vi "Requests.vi"(8 "error in (no error)":errorcluster, 9 "write enable":bool=TRUE, 11 "SMSD in":refnum<class "SMSD-DI.lvclass">) -> (0 "error out":errorcluster, 3 "SMSD out":refnum<class "SMSD-DI.lvclass">)   [LabVIEW 2019, in "SMSD-DI.lvclass"]
uses:
  SMSD-DI.lvclass
  D:/my_projects/projects/Algorithms/Labview/19/Modbus/MB_TCP2/MB_TCP.lvclass
  D:/my_projects/projects/Algorithms/Labview/19/Modbus/MB_TCP2/SMSD/SMSD.lvclass
  MB_TCP.lvclass/MB_TCP.ctl
  Ctl/ERROR_OR_COMMANT_Type.ctl
  SMSD.lvclass/SMSD.ctl
  NI_modbus_upd/TCP/TCP.lvclass/TCP.ctl
  SMSD_cmd_format.vi
  NI_modbus_upd/TCP/Protocol Read.vi
  NI_modbus_upd/TCP/Protocol Write.vi
  Data Access/Read TCP.vi
  SMSD_cmd_Data_format.vi
  SMSD_LAN_COMMAND.vi
  <vilib>/Utility/error.llb/Clear Errors.vi
  SMSD.lvclass
  NI_modbus_upd/TCP/TCP.lvclass
  ICPCON Registers/ICPCON Registers.lvlib
  MB_TCP.lvclass
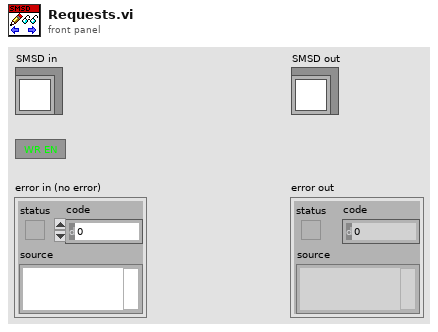
[diagram p1: front panel]
types:
  T1 = enum8{"CMD_PowerSTEP01_END", "CMD_PowerSTEP01_GET_SPEED", "CMD_PowerSTEP01_STATUS_IN_EVENT", "CMD_PowerSTEP01_SET_MODE", "CMD_PowerSTEP01_GET_MODE", "CMD_PowerSTEP01_SET_MIN_SPEED", "CMD_PowerSTEP01_SET_MAX_SPEED", "CMD_PowerSTEP01_SET_ACC", "CMD_PowerSTEP01_SET_DEC", "CMD_PowerSTEP01_SET_FS_SPEED", "CMD_PowerSTEP01_SET_MASK_EVENT", "CMD_PowerSTEP01_GET_ABS_POS", "CMD_PowerSTEP01_GET_EL_POS", "CMD_PowerSTEP01_GET_STATUS_AND_CLR", "CMD_PowerSTEP01_RUN_F", "CMD_PowerSTEP01_RUN_R", "CMD_PowerSTEP01_MOVE_F", "CMD_PowerSTEP01_MOVE_R", "CMD_PowerSTEP01_GO_TO_F", "CMD_PowerSTEP01_GO_TO_R", "CMD_PowerSTEP01_GO_UNTIL_F", "CMD_PowerSTEP01_GO_UNTIL_R", "CMD_PowerSTEP01_SCAN_ZERO_F", "CMD_PowerSTEP01_SCAN_ZERO_R", "CMD_PowerSTEP01_SCAN_LABEL_F", "CMD_PowerSTEP01_SCAN_LABEL_R", "CMD_PowerSTEP01_GO_ZERO", "CMD_PowerSTEP01_GO_LABEL", "CMD_PowerSTEP01_GO_TO", "CMD_PowerSTEP01_RESET_POS", "CMD_PowerSTEP01_RESET_POWERSTEP01", "CMD_PowerSTEP01_SOFT_STOP", "CMD_PowerSTEP01_HARD_STOP", "CMD_PowerSTEP01_SOFT_HI_Z", "CMD_PowerSTEP01_HARD_HI_Z", "CMD_PowerSTEP01_SET_WAIT", "CMD_PowerSTEP01_SET_RELE", "CMD_PowerSTEP01_CLR_RELE", "CMD_PowerSTEP01_GET_RELE", "CMD_PowerSTEP01_WAIT_IN0", "CMD_PowerSTEP01_WAIT_IN1", "CMD_PowerSTEP01_GOTO_PROGRAM", "CMD_PowerSTEP01_GOTO_PROGRAM_IF_IN0", "CMD_PowerSTEP01_GOTO_PROGRAM_IF_IN1", "CMD_PowerSTEP01_LOOP_PROGRAM", "CMD_PowerSTEP01_CALL_PROGRAM", "CMD_PowerSTEP01_RETURN_PROGRAM", "CMD_PowerSTEP01_START_PROGRAM_MEM0", "CMD_PowerSTEP01_START_PROGRAM_MEM1", "CMD_PowerSTEP01_START_PROGRAM_MEM2", "CMD_PowerSTEP01_START_PROGRAM_MEM3", "CMD_PowerSTEP01_STOP_PROGRAM_MEM", "CMD_PowerSTEP01_STEP_CLOCK", "CMD_PowerSTEP01_STOP_USB", "CMD_PowerSTEP01_GET_MIN_SPEED", "CMD_PowerSTEP01_GET_MAX_SPEED", "CMD_PowerSTEP01_GET_STACK", "CMD_PowerSTEP01_GOTO_PROGRAM_IF_ZERO", "CMD_PowerSTEP01_GOTO_PROGRAM_IF_IN_ZERO", "CMD_PowerSTEP01_WAIT_CONTINUE", "CMD_PowerSTEP01_SET_WAIT_2", "CMD_PowerSTEP01_SCAN_MARK2_F", "CMD_PowerSTEP01_SCAN_MARK2_R"}
  T2 = typedef "SMSD.lvclass/ERROR_OR_COMMANT_Type.ctl" = enum8{"OK", "OK_ACCESS", "ERROR_ACCESS", "ERROR_ACCESS_TIMEOUT", "ERROR_XOR", "ERROR_NO_COMMAND", "ERROR_LEN", "ERROR_RANGE", "ERROR_WRITE", "ERROR_READ", "ERROR_PROGRAMS", "ERROR_WRITE_SETUP", "NO_NEXT", "END_PROGRAMS", "COMMAND_GET_STATUS_IN_EVENT", "COMMAND_GET_MODE", "COMMAND_GET_ABS_POS", "COMMAND_GET_EL_POS", "COMMAND_GET_SPEED", "COMMAND_GET_MIN_SPEED", "COMMAND_GET_MAX_SPEED", "COMMAND_GET_STACK", "STATUS_RELE_SET", "STATUS_RELE_CLR"}
  T3 = typedef "ICPCON Registers.lvlib/ICPCON Data.ctl" = cluster{"UTF":refnum<data-value>, "DI":refnum<data-value>, "DW":refnum<data-value>, "DO":refnum<data-value>, "IR":refnum<data-value>, "WR":refnum<data-value>, "OR":refnum<data-value>, "modified":refnum<data-value>}
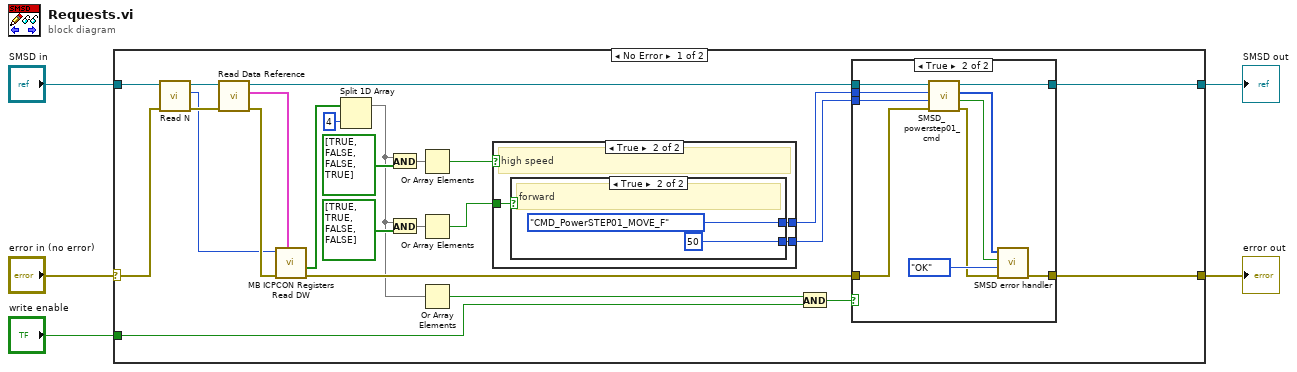
[diagram p0: block diagram]
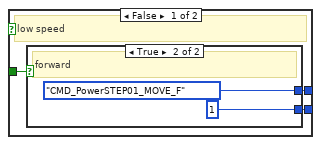
[diagram p2: hidden frame]
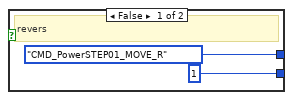
[diagram p3: hidden frame]
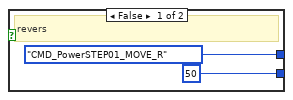
[diagram p4: hidden frame]
diagram:
  n1 = case shown="No Error" "error in (no error)" {
    selector: "error in (no error)" -> [w6 w58]
    tunnel: [w28 w58] -> w1
    tunnel: [w30 w57] -> w2
    tunnel: "SMSD in" -> [w11 w57]
    tunnel: "write enable" -> [w15 _]
    frame No Error {
      n2 = call "Read N.vi"("error in (no error)"=w6, "MB_TCP in"=w11) -> ("error out"=w12:errorcluster, "N"=w7:i32, "MB_TCP out"=w13:refnum<class "SMSD-DI.lvclass">)  [unwired: 7 in]
      n3 = call "Read Data Reference.vi"("error in (no error)"=w12, "MB_TCP in"=w13) -> ("error out"=w8:errorcluster, "Data"=w9:T3, "MB_TCP out"=w10:refnum<class "SMSD-DI.lvclass">)  [unwired: 7 in]
      n4 = call "MB ICPCON Registers Read DW.vi"("Data Reference"=w9, "error in (no error)"=w8, "N"=w7) -> ("error out"=w29:errorcluster, "Bits out"=w26:bool[])  [unwired: 7 in]
      n5 = Split 1D Array(array=w26, index=4) -> (first subarray=w21:bool[])  [unwired: 1 out]
      n6 = And(x=w21, y=bool[] [TRUE, FALSE, FALSE, TRUE] ("x")) -> (x .and. y?=w25:bool[])
      n7 = And(x=w21, y=bool[] [TRUE, TRUE, FALSE, FALSE] ("x")) -> (x .and. y?=w22:bool[])
      n8 = Or Array Elements(Boolean array=w25) -> (logical OR=w20:bool)
      n9 = Or Array Elements(Boolean array=w22) -> (logical OR=w19:bool)
      n10 = Or Array Elements(Boolean array=w21) -> (logical OR=w14:bool)
      n11 = case shown="True" w20 {
        tunnel: w19 -> [w33 w40]
        tunnel: [w32 w39] -> w18
        tunnel: [w31 w38] -> w17
        frame False {
          # "low speed"
          n12 = case shown="True" w33 {
            tunnel: [T1."CMD_PowerSTEP01_MOVE_R" ("COMMAND (END)") T1."CMD_PowerSTEP01_MOVE_F" ("COMMAND (END)")] -> w32
            tunnel: [u32 1 ("DATA (0)") u32 1 ("DATA (0)")] -> w31
            frame False {
              # "revers"
            }
            frame True {
              # "forward"
            }
          }
        }
        frame True {
          # "high speed"
          n13 = case shown="True" w40 {
            tunnel: [T1."CMD_PowerSTEP01_MOVE_R" ("COMMAND (END)") T1."CMD_PowerSTEP01_MOVE_F" ("COMMAND (END)")] -> w39
            tunnel: [u32 50 ("DATA (0)") u32 50 ("DATA (0)")] -> w38
            frame False {
              # "revers"
            }
            frame True {
              # "forward"
            }
          }
        }
      }
      n14 = And(x=w14, y=w15) -> (x .and. y?=w16:bool)
      n15 = case shown="True" w16 {
        tunnel: [w46 w56] -> w30
        tunnel: w10 -> [w46 w55]
        tunnel: [w45 w50] -> w28
        tunnel: w29 -> [w45 w49]
        tunnel: w18 -> [_ w48]
        tunnel: w17 -> [_ w47]
        frame False {
        }
        frame True {
          n16 = call "SMSD_powerstep01_cmd.vi"("error in (no error)"=w49, "DATA (0)"=w47, "COMMAND (END)"=w48, "SMSD in"=w55) -> ("error out"=w51:errorcluster, "timed out?"=w52:bool, "data"=w54:u8[], "SMSD out"=w56:refnum<class "SMSD-DI.lvclass">)  [unwired: 4 in]
          n17 = call "SMSD error handler.vi"("error in (no error)"=w51, "correct answer (OK)"=ERROR_OR_COMMANT_Type."OK" ("coerced x 2"), "timed out?"=w52, "data"=w54) -> ("error out"=w50:errorcluster)  [unwired: 7 in]
        }
      }
    }
    frame Error {
    }
  }
  "error out" <- w1
  "SMSD out" <- w2
